vi "Configure Range.vi"(5 "Calculate Block (1: Calculate Block 1)":i32(ring)=1 items=["Calculate Block 1"=1, "Calculate Block 2"=2, "Calculate Block 3"=3, "Calculate Block 4"=4], 6 "Power Range (0: Lower Range)":i32(ring) items=["Lower Range", "Upper Range"], 7 "Auto Range (T: Enable)":bool=TRUE, 8 "error in (no error)":errorcluster, 9 "Upper Limit (90 dBm)":dbl=90.0, 10 "Lower Limit (-90 dBm)":dbl=-90.0, 11 "VISA resource name":refnum<visa-resource-name>) -> (0 "error out":errorcluster, 3 "VISA resource name out":refnum<visa-resource-name>)   [LabVIEW 2018, in "Agilent U2000 Series.lvlib"]
doc: "Configures the instrument's ranging capabilities. Enabling auto ranging allows the instrument to choose its own range. Otherwise, custom limits can be used to set up the range. Should the range be exceeded, the result can be known by calling the Query Range Test VI."
uses:
  Agilent U2000 Series.lvlib
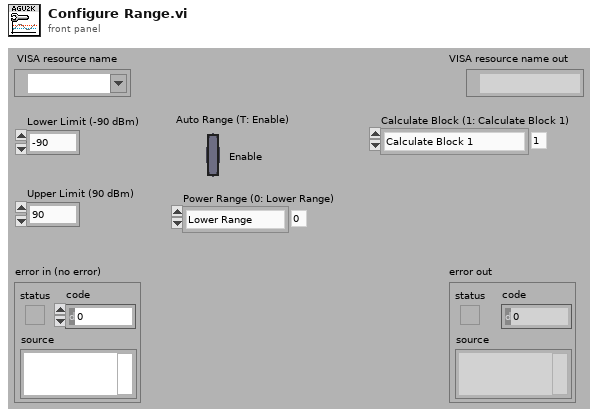
[diagram p1: front panel]
types:
  T1 = typedef "Agilent U2000 Series.lvlib/Extended User Data.ctl" = cluster{"U2000 Series Mode":u16, "Trigger Source Int/Ext":bool}
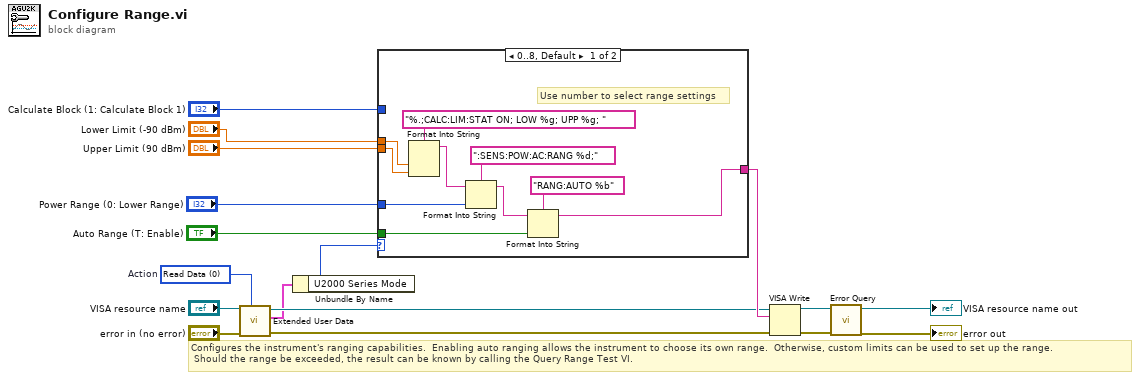
[diagram p0: block diagram]
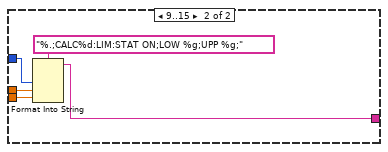
[diagram p2: hidden frame]
diagram:
  w3 = 0 items=["Read Data", "Write Data", "Clear Data", "Clear ALL Data"]  # Action
  # "Configures the instrument's ranging capabilities.  Enabling auto ranging allows the instrument to choose its own range.  Otherwise, custom limits can be used to set up the range. \n Should the range be exceeded, the result can be known by calling the Query Range Test VI."
  n1 = call "Extended User Data.vi"("Action (1: Write Data)"=w3, "error in (no error)"="error in (no error)", "VISA resource name"="VISA resource name") -> ("error out"=w4:errorcluster, "User Data Out"=w2:T1, "VISA resource name out"=w5:refnum<visa-resource-name>)  [unwired: 1 in, 5 out]
  n2 = Unbundle By Name(w2) -> ("U2000 Series Mode"=w1:u16)
  n3 = case shown="0..8, Default" w1 {
    tunnel: "Lower Limit (-90 dBm)" -> [w27 w31]
    tunnel: "Upper Limit (90 dBm)" -> [w26 w30]
    tunnel: "Calculate Block (1: Calculate Block 1)" -> [_ w29]
    tunnel: [w20 w28] -> w10
    tunnel: "Power Range (0: Lower Range)" -> [w19 _]
    tunnel: "Auto Range (T: Enable)" -> [w18 _]
    frame 0..8, Default {
      # "Use number to select range settings"
      n4 = Format Into String(format string="%.;CALC:LIM:STAT ON; LOW %g; UPP %g; ", w27, w26) -> (resulting string=w24:string)  [unwired: 2 in, 1 out]
      n5 = Format Into String(format string=":SENS:POW:AC:RANG %d;", initial string=w24, w19) -> (resulting string=w22:string)  [unwired: 1 in, 1 out]
      n6 = Format Into String(format string="RANG:AUTO %b", initial string=w22, w18) -> (resulting string=w20:string)  [unwired: 1 in, 1 out]
    }
    frame 9..15 {
      n7 = Format Into String(format string="%.;CALC%d:LIM:STAT ON;LOW %g;UPP %g;", w29, w31, w30) -> (resulting string=w28:string)  [unwired: 2 in, 1 out]
    }
  }
  n8 = VISA Write(VISA resource name=w5, write buffer=w10, error in (no error)=w4) -> (VISA resource name out=w17:refnum<visa-resource-name>, error out=w16:errorcluster)  [unwired: 1 out]
  n9 = call "Error Query.vi"("error in (no error)"=w16, "VISA resource name"=w17) -> ("error out"=→"error out":errorcluster, "VISA resource name out"=→"VISA resource name out":refnum<visa-resource-name>)  [unwired: 8 out]
